vi "Speech Recognition Text Callback.vi"(4 "Front Panel Objects":T1, 5 "Event Data":cluster{"sender":refnum<k24>, "e":refnum<k24>}, 6 "Control Ref":refnum<k24>, 7 "Event Common Data":T2) -> ()   [LabVIEW 2017]
uses:
  System.Speech
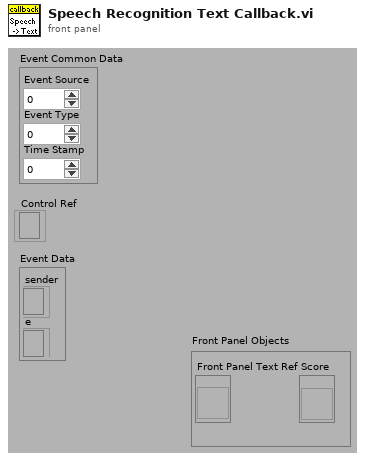
[diagram p1: front panel]
types:
  T1 = cluster{"Front Panel Text Ref":refnum<vi>, "Score":refnum<vi>}
  T2 = cluster{"Event Source":i32, "Event Type":u32, "Time Stamp":u32}
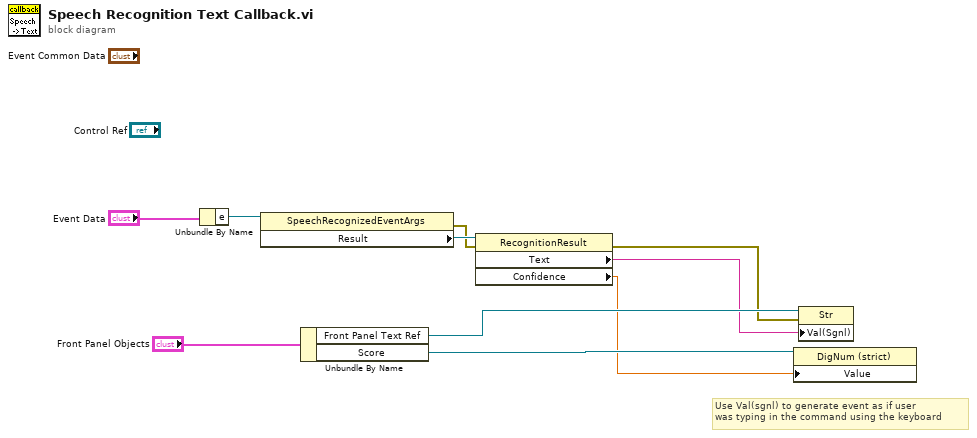
[diagram p0: block diagram]
diagram:
  # "Use Val(sgnl) to generate event as if user\nwas typing in the command using the keyboard"
  n1 = Unbundle By Name("Event Data") -> ("e"=w9:refnum<k24>)
  n2 = property class="SpeechRecognizedEventArgs"(reference=w9) -> (error out=w7:errorcluster, "Result"=w8:refnum<k24>)  [unwired: 1 in, 1 out]
  n3 = Unbundle By Name("Front Panel Objects") -> ("Front Panel Text Ref"=w5:refnum<vi>, "Score"=w4:refnum<vi>)
  n4 = property class="RecognitionResult"(reference=w8, error in=w7) -> (error out=w2:errorcluster, "Text"=w1:string, "Confidence"=w3:sgl)  [unwired: 1 out]
  n5 = property class="DigNum (strict)"(reference=w4, "Value"=w3) -> ()  [unwired: 1 in, 2 out]
  n6 = property class="Str"(reference=w5, error in=w2, "Val(Sgnl)"=w1) -> ()  [unwired: 2 out]
